vi "stop.vi"(0 "HGF_TaskLoop in":refnum<class "HGF_TaskLoop.lvclass">, 5 "error in (no error)":errorcluster) -> (14 "HGF_TaskLoop out":refnum<class "HGF_TaskLoop.lvclass">, 19 "error out":errorcluster)   [LabVIEW 2014, in "HGF_BaseClasses.lvlib" / "HGF_TaskLoop.lvclass"]
doc: "Call TaskDeinitialize from all member objects\n\nF.Berck@gsi.de\nGSI Darmstadt 2010"
uses:
  HGF_TaskLoop.lvclass
  HGF_ThreadTask/HGF_ThreadTask.lvclass
  HGF_Visitable/HGF_Visitable.lvclass
  HGF_Event/HGF_Event.lvclass
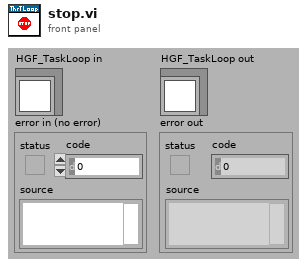
[diagram p1: front panel]
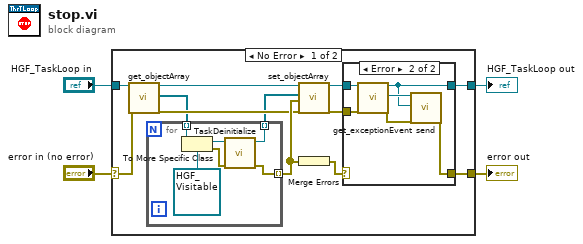
[diagram p0: block diagram]
diagram:
  n1 = case shown="No Error" "error in (no error)" {
    selector: "error in (no error)" -> [w6 w32]
    tunnel: [w5 w32] -> w3
    tunnel: [w7 w31] -> w1
    tunnel: "HGF_TaskLoop in" -> [w8 w31]
    frame No Error {
      n2 = call "get_objectArray.vi"("HGF_ThreadTask"=w8, "error in (no error)"=w6) -> ("dup HGF_ThreadTask"=w9:refnum<class "HGF_TaskLoop.lvclass">, "objectArray"=w10:refnum<class>[], "error out"=w12:errorcluster)  [unwired: 15 out]
      n3 = for {
        tunnel: [w25] -> w13 mode=indexing
        tunnel: w10 -> [w29] mode=indexing
        tunnel: [w27] -> w11 mode=indexing
        n4 = To More Specific Class(target class=refnum<class "HGF_Visitable.lvclass"> refnum ("HGF_BaseClasses.lvlib:HGF_Visitable.lvclass"), reference=w29) -> (specific class reference=w28:refnum<class "HGF_Visitable.lvclass">, error out=w26:errorcluster)  [unwired: 1 in]
        n5 = call-dynamic "TaskDeinitialize.vi"("error in (no error)"=w26, "HGF_Visitable in"=w28) -> ("error out"=w25:errorcluster, "HGF_Visitable out"=w27:refnum<class "HGF_Visitable.lvclass">)  [unwired: 8 in]
      }
      n6 = call "set_objectArray.vi"("HGF_ThreadTask"=w9, "objectArray"=w11, "errorArray"=w13, "error in (no error)"=w12) -> ("dup HGF_ThreadTask"=w14:refnum<class "HGF_TaskLoop.lvclass">, "error out"=w15:errorcluster)  [unwired: 14 out]
      n7 = Merge Errors(w13) -> (w16:errorcluster)
      n8 = case shown="Error" w16 {
        tunnel: w14 -> [w18 w24]
        tunnel: [w18 w19] -> w7
        tunnel: w15 -> [w17 w23]
        tunnel: [w17 w20] -> w5
        frame No Error {
        }
        frame Error {
          n9 = call "get_exceptionEvent.vi"("HGF_ThreadTask"=w24, "error in (no error)"=w23) -> ("dup HGF_ThreadTask"=w19:refnum<class "HGF_TaskLoop.lvclass">, "exceptionEvent"=w22:refnum<class "HGF_Event.lvclass">, "error out"=w21:errorcluster)  [unwired: 15 out]
          n10 = call-dynamic "send.vi"("HGF_Event"=w22, "Object"=w19, "error in (no error)"=w21) -> ("error out"=w20:errorcluster)  [unwired: 2 in, 14 out]
        }
      }
    }
    frame Error {
    }
  }
  "error out" <- w3
  "HGF_TaskLoop out" <- w1
